vi "readt.vi"(8 "error in":errorcluster, 10 "Boolean":bool) -> (0 "error out":errorcluster, 2 "appended array":dbl[](array[numeric]))   [LabVIEW 2015]
uses:
  <vilib>/Analysis/baseanly.llb/Mean (DBL).vi
  <vilib>/Analysis/NI_AALBase.lvlib
panel:
  out "subarray":dbl[](array[numeric])
  out "Array":dbl[][](array[numeric])
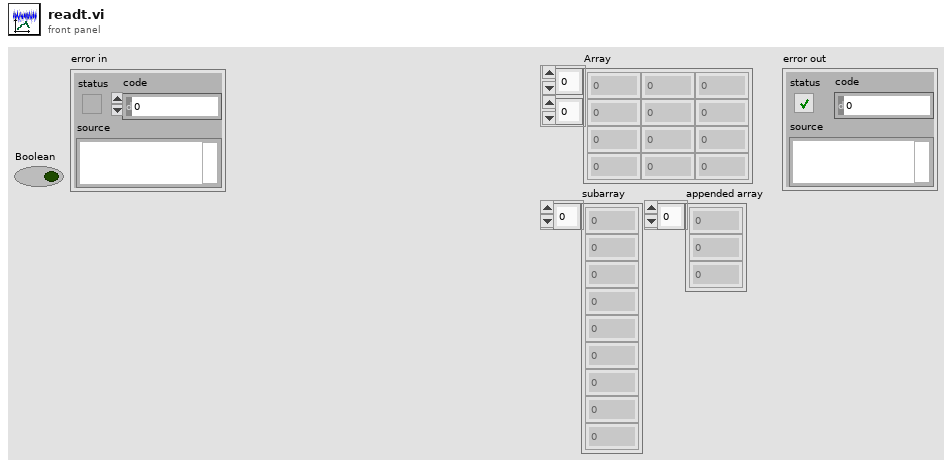
[diagram p1: front panel]
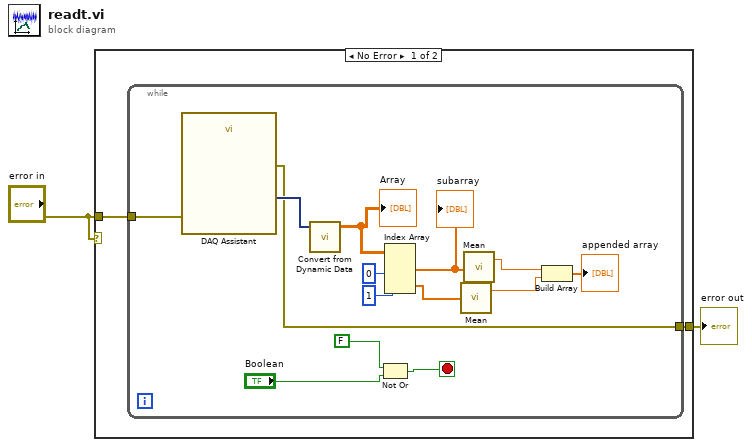
[diagram p0: block diagram]
diagram:
  n1 = case shown="No Error" "error in" {
    tunnel: "error in" -> [w4 w19]
    tunnel: [w3 w19] -> w2
    frame No Error {
      n2 = while {
        tunnel: [w6] -> w3
        tunnel: w4 -> [w5]
        stop <- w7 stop-if-true
        n3 = call "DAQ Assistant"("error in"=w5) -> ("data"=w18:dynamicdata, "error out"=w6:errorcluster)  [unwired: 16 in, 1 out]
        n4 = call "Convert from Dynamic Data"("Dynamic Data Type"=w18) -> ("Array"=w17:dbl[][])  [unwired: 3 in]
        "Array" <- w17
        n5 = Not Or(1:"Boolean", 2:FALSE) -> (0:w7:bool)
        n6 = Index Array(array=w17, index (col) #1=0 ("disabled index (col)"), index (col) #2=1 ("index (col)")) -> (element #1=w16:dbl[], element #2=w13:dbl[])  [unwired: 2 in]
        "subarray" <- w16
        n7 = call-poly <vilib>:"Mean.vi"("X"=w13) -> ("mean"=w11:dbl)  [unwired: 1 out]
        n8 = call-poly <vilib>:"Mean.vi"("X"=w16) -> ("mean"=w12:dbl)  [unwired: 1 out]
        n9 = Build Array(w12, w11) -> (→"appended array":dbl[])
      }
    }
    frame Error {
    }
  }
  "error out" <- w2
